vi "PID-Parameter Druckregler einstellen optional.vi"() -> ()   [LabVIEW 2020, in "Erweiterte Konfig.lvlib"]
uses:
  Erweiterte Konfig.lvlib
  Visualisierungs Elemente/Button.ctl
  Visualisierungs Elemente/Zahlen-Eingabefeld.ctl
  Visualisierungs Elemente/Zahlen-Ausgabefeld.ctl
  <vilib>/Utility/miscctls.llb/LVPositionTypeDef.ctl
  cRIO/PC/Aktionen FGV Druckregler.ctl
  cRIO/PC/Kommunikation mit cRIO.lvlib
  Allgemein/allgemeine Sub-VIs.lvlib
  Sprachverwaltung/Sprachverwaltung.lvlib
panel:
  in  "Nach rechts":bool
  in  "Nach links 2":bool
  in  "Nach rechts 2":bool
  in  "Nach links":bool
  in  "Gaskühler Regler -":T1 caption="Ausgang Regler -" format="%#_5g"
  in  "Gaskühler Regler +":T1 caption="Ausgang Regler +" format="%#_5g"
  in  "Gaskühler D":T1 caption="Ausgang D" format="%#_5g"
  in  "Gaskühler I":T1 caption="Ausgang I" format="%#_5g"
  in  "Gaskühler P":T1 caption="Ausgang P" format="%#_5g"
  in  "Gaskühler Regler Toleranz":bool caption="Ausgang Regler Toleranz"
  out "Gaskühler Sollwert":T2 caption="Ausgang Sollwert" format="%.1f"
  out "Gaskühler Istwert":T2 caption="Ausgang Istwert" format="%.1f"
  out "Gaskühler Regler Ausgang":T2 caption="Ausgang Regler Ausgang" format="%.2f"
  out "Gaskühler Analog Ausgang":T2 caption="Ausgang Analog Ausgang" format="%.2f"
  out "Gaskühler Integral":T2 caption="Ausgang Integral" format="%.2f"
  out "Gaskühler Derivative":T2 caption="Ausgang Derivative" format="%.2f"
  out "Gaskühler":sgl[][](graph) caption="Ausgang"
  in  "Druck Kalter Block Regler -":T1 caption="Ausgang Regler -" format="%#_5g"
  in  "Druck Kalter Block Regler +":T1 caption="Ausgang Regler +" format="%#_5g"
  in  "Druck Kalter Block D":T1 caption="Ausgang D" format="%#_5g"
  in  "Druck Kalter Block I":T1 caption="Ausgang I" format="%#_5g"
  in  "Druck Kalter Block P":T1 caption="Ausgang P" format="%#_5g"
  in  "Druck Kalter Block Regler Toleranz":bool caption="Ausgang Regler Toleranz"
  out "Druck Kalter Block Sollwert":T2 caption="Ausgang Sollwert" format="%.1f"
  out "Druck Kalter Block Istwert":T2 caption="Ausgang Istwert" format="%.1f"
  out "Druck Kalter Block Regler Ausgang":T2 caption="Ausgang Regler Ausgang" format="%.2f"
  out "Druck Kalter Block Analog Ausgang":T2 caption="Ausgang Analog Ausgang" format="%.2f"
  out "Druck Kalter Block Integral":T2 caption="Ausgang Integral" format="%.2f"
  out "Druck Kalter Block Derivative":T2 caption="Ausgang Derivative" format="%.2f"
  out "Druck Kalter Block":sgl[][](graph) caption="Ausgang"
  out "Pumpe":sgl[][](graph)
  out "Pumpe Derivative":T2 format="%.2f"
  out "Pumpe Integral":T2 format="%.2f"
  out "Pumpe Analog Ausgang":T2 format="%.2f"
  out "Pumpe Regler Ausgang":T2 format="%.2f"
  out "Pumpe Istwert":T2 format="%.1f"
  out "Pumpe Sollwert":T2 format="%.1f"
  in  "Pumpe Regler -":T1 format="%#_5g"
  in  "Pumpe Regler +":T1 format="%#_5g"
  in  "Pumpe D":T1 format="%#_5g"
  in  "Pumpe I":T1 format="%#_5g"
  in  "Pumpe P":T1 format="%#_5g"
  in  "Pumpe Regler Toleranz":bool
  in  "BEENDEN":T3
  in  "Ausgang Regler -":T1 format="%#_5g"
  in  "Ausgang Regler +":T1 format="%#_5g"
  in  "Ausgang D":T1 format="%#_5g"
  in  "Ausgang I":T1 format="%#_5g"
  in  "Ausgang P":T1 format="%#_5g"
  in  "Ausgang Regler Toleranz":bool
  out "Ausgang Sollwert":T2 format="%.1f"
  out "Ausgang Istwert":T2 format="%.1f"
  out "Ausgang Regler Ausgang":T2 format="%.2f"
  out "Ausgang Analog Ausgang":T2 format="%.2f"
  out "Ausgang Integral":T2 format="%.2f"
  out "Ausgang Derivative":T2 format="%.2f"
  out "Ausgang":sgl[][](graph)
  out "FT-IR":sgl[][](graph)
  out "FT-IR Sollwert":T2 format="%.2f"
  out "FT-IR Istwert":T2 format="%.2f"
  out "FT-IR Regler Ausgang":T2 format="%.2f"
  out "FT-IR Analog Ausgang":T2 format="%.2f"
  out "FT-IR Integral":T2 format="%.2f"
  out "FT-IR Derivative":T2 format="%.2f"
  in  "FT-IR Regler -":T1 format="%#_5g"
  in  "FT-IR Regler +":T1 format="%#_5g"
  in  "FT-IR D":T1 format="%#_5g"
  in  "FT-IR I":T1 format="%#_5g"
  in  "FT-IR P":T1 format="%#_5g"
  in  "FT-IR Regler Toleranz":bool
  # "Parameters Pressure Controller"
  # "Pressure Inlet"
  # "Druck Kalter Block"
  # "Pressure Outlet"
  # "Flow (Pump)"
  # "Gaskühler"
  # "Setpoint:"
  # "Setpoint:"
  # "Setpoint:"
  # "Setpoint:"
  # "Setpoint:"
  # "Intensification KR:"
  # "Intensification KR:"
  # "Intensification KR:"
  # "Intensification KR:"
  # "Intensification KR:"
  # "Actual:"
  # "Actual:"
  # "Actual:"
  # "Actual:"
  # "Actual:"
  # "Reset time TN:"
  # "Reset time TN:"
  # "Reset time TN:"
  # "Reset time TN:"
  # "sec"
  # "sec"
  # "sec"
  # "sec"
  # "Reset time TN:"
  # "sec"
  # "Controller OUT:"
  # "Controller OUT:"
  # "Controller OUT:"
  # "Controller OUT:"
  # "Controller OUT:"
  # "Analog OUT:"
  # "Analog OUT:"
  # "Analog OUT:"
  # "Analog OUT:"
  # "Analog OUT:"
  # "Derivative time TD:"
  # "Derivative time TD:"
  # "Derivative time TD:"
  # "Derivative time TD:"
  # "Derivative time TD:"
  # "sec"
  # "sec"
  # "sec"
  # "sec"
  # "sec"
  # "Intagral Action:"
  # "Intagral Action:"
  # "Intagral Action:"
  # "Intagral Action:"
  # "Intagral Action:"
  # "Derivative Action:"
  # "Derivative Action:"
  # "Derivative Action:"
  # "Derivative Action:"
  # "Derivative Action:"
  # "Contr. tolerance +:"
  # "Contr. tolerance +:"
  # "Contr. tolerance +:"
  # "Contr. tolerance +:"
  # "mbar"
  # "mbar"
  # "Contr. tolerance +:"
  # "l/min"
  # "°C"
  # "mbar"
  # "Contr. tolerance - :"
  # "Contr. tolerance - :"
  # "Contr. tolerance - :"
  # "l/min"
  # "Contr. tolerance - :"
  # "mbar"
  # "mbar"
  # "Contr. tolerance - :"
  # "mbar"
  # "°C"
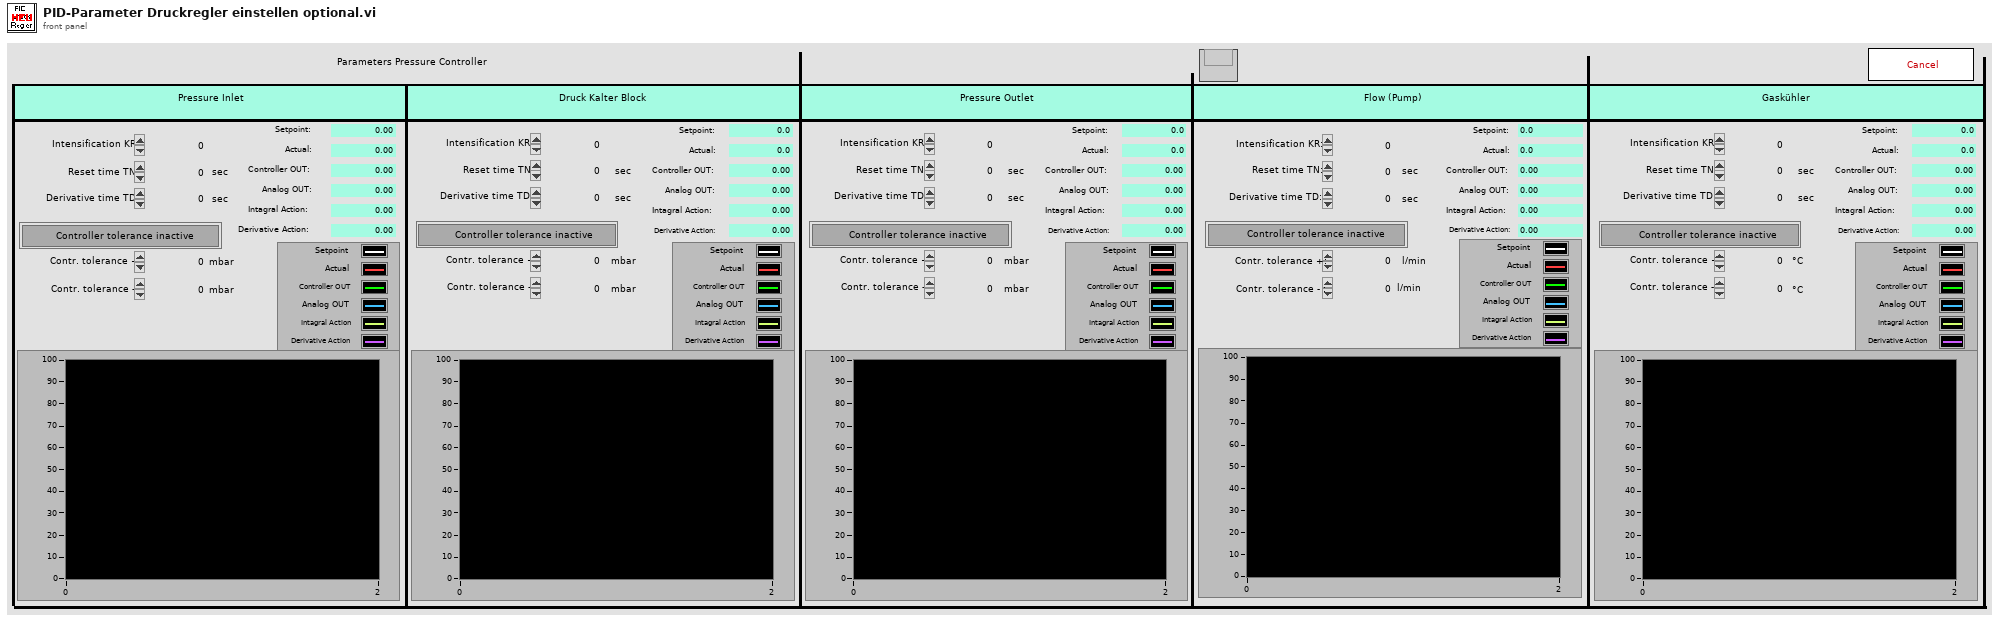
[diagram p1: front panel]
types:
  T1 = typedef "Zahlen-Eingabefeld.ctl" = sgl
  T2 = typedef "Zahlen-Ausgabefeld.ctl" = sgl
  T3 = typedef "Button.ctl" = bool
  T4 = typedef "LVPositionTypeDef.ctl" = cluster{"Left":i32, "Top":i32}
  T5 = typedef "Kommunikation mit cRIO.lvlib/Aktionen FGV Druckregler.ctl" = enum16{"lesen", "Parameter", "Istwerte"}
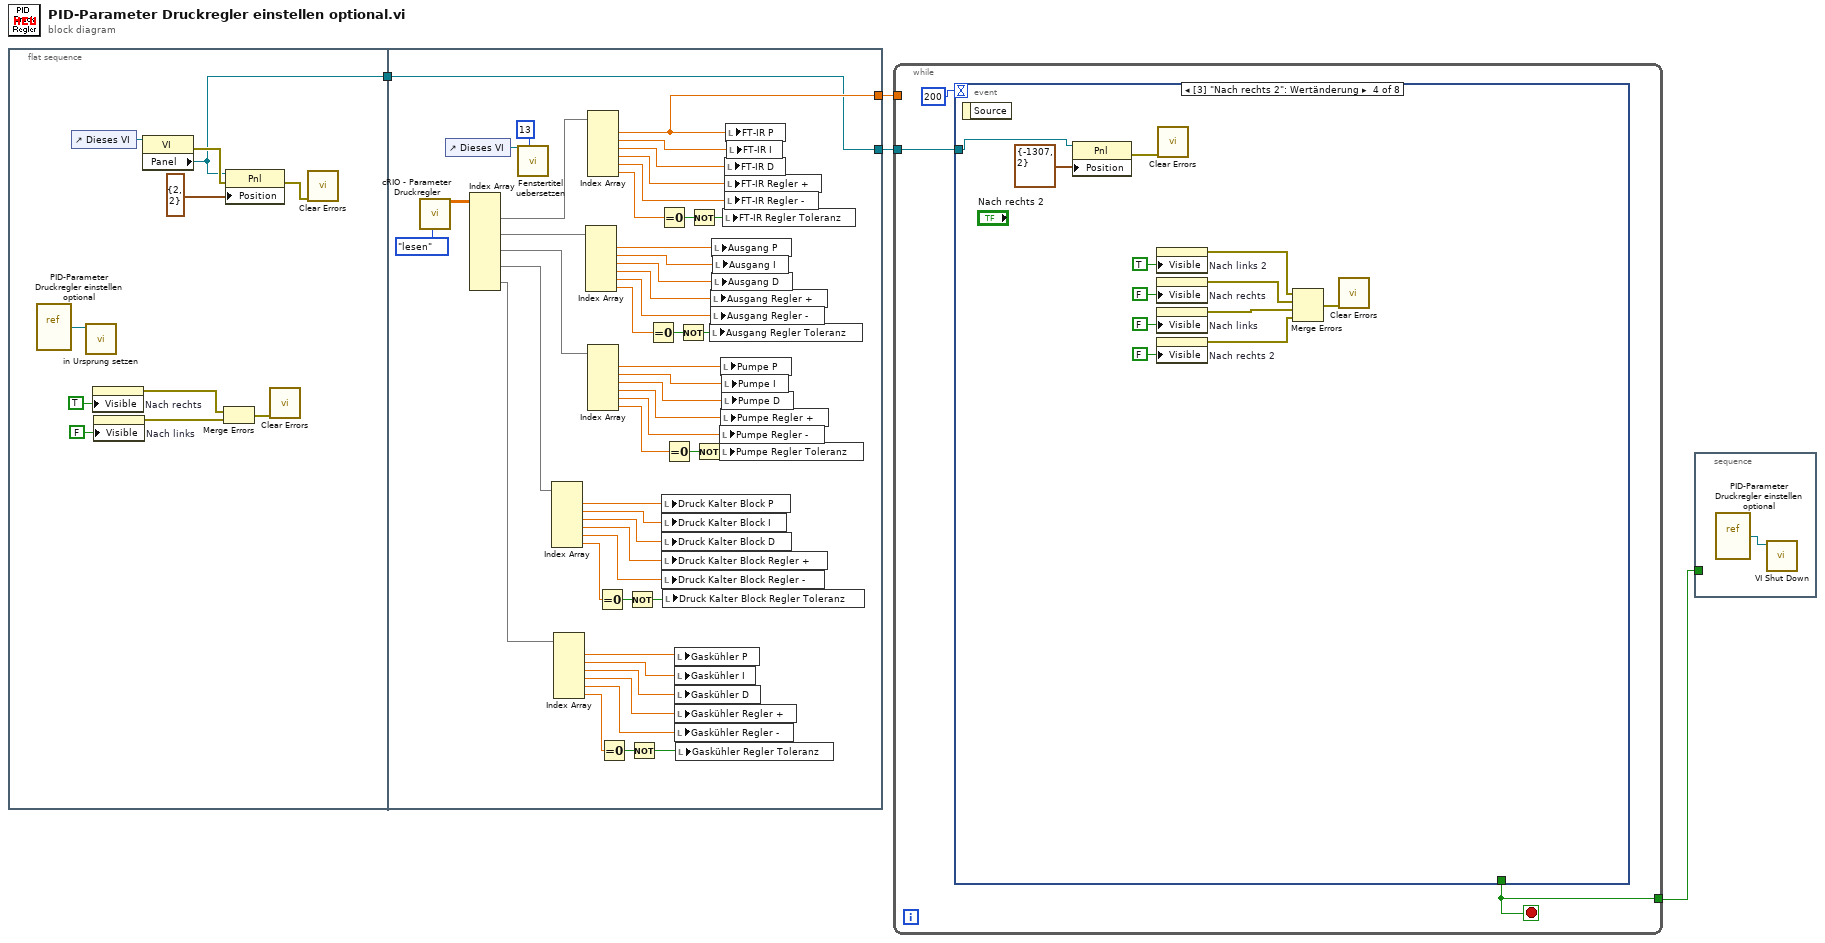
[diagram p0: block diagram]
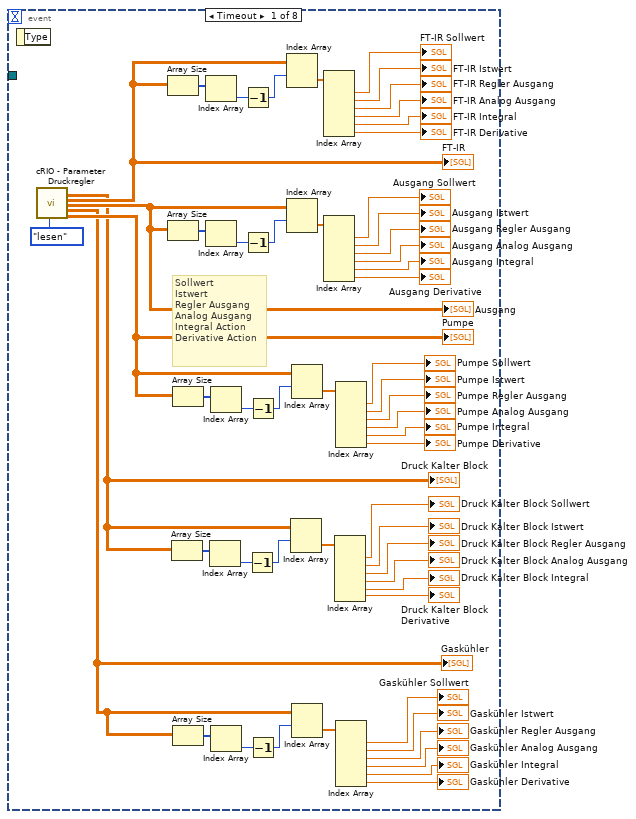
[diagram p2: hidden frame]
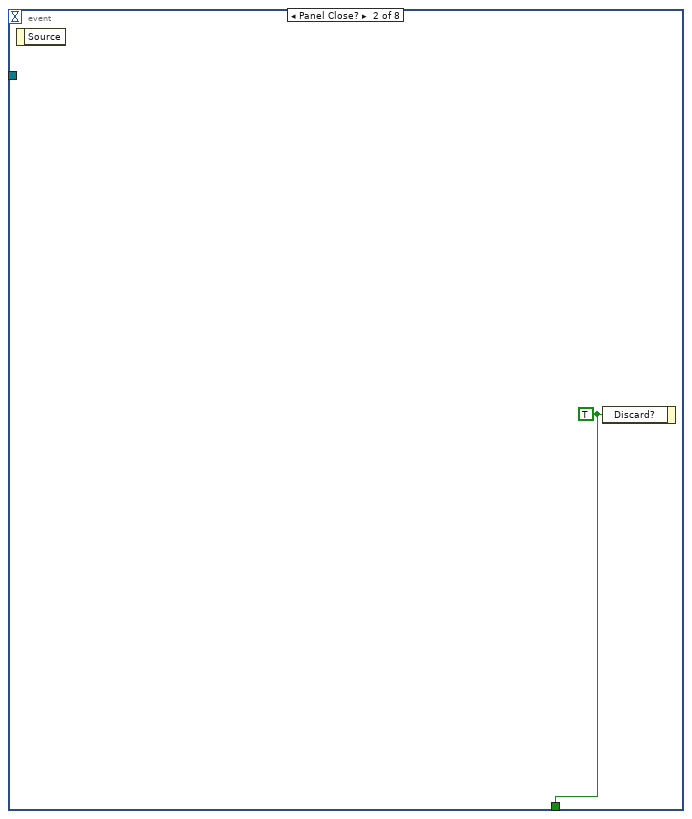
[diagram p3: hidden frame]
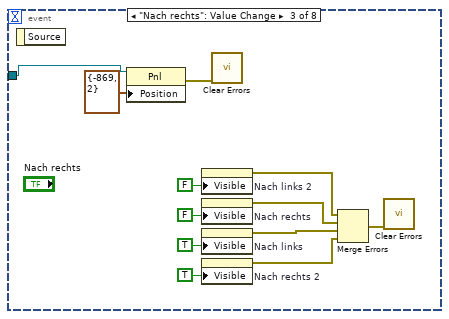
[diagram p4: hidden frame]
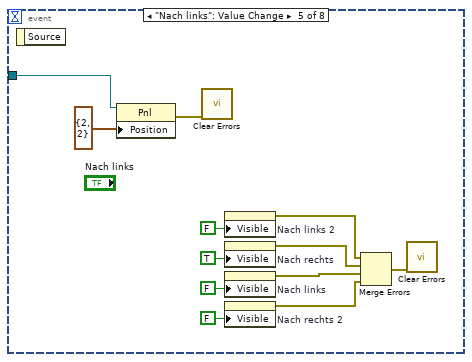
[diagram p5: hidden frame]
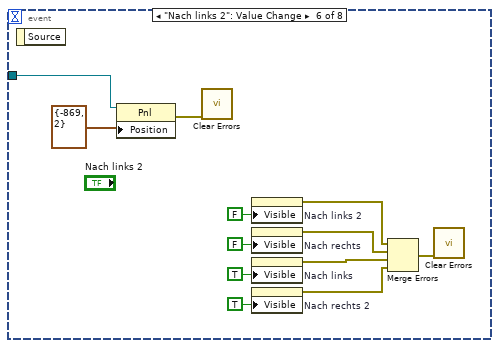
[diagram p6: hidden frame]
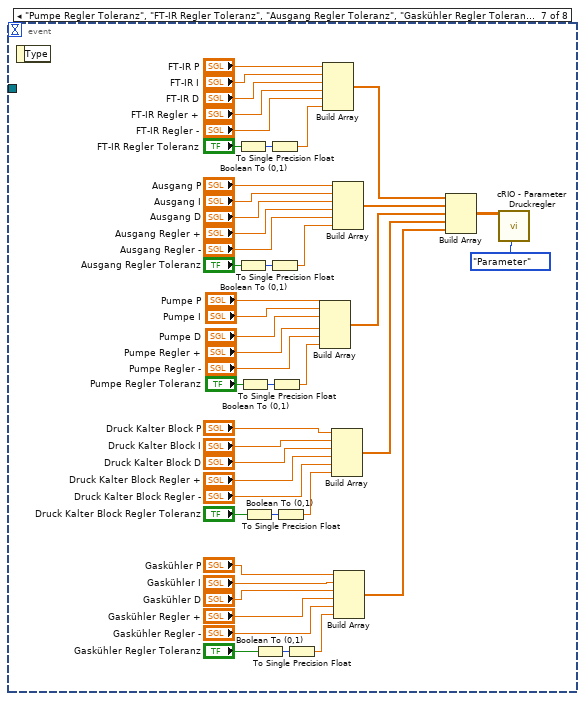
[diagram p7: hidden frame]
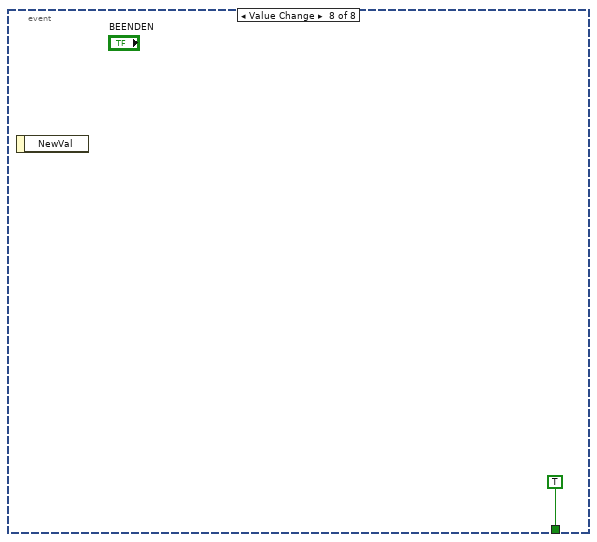
[diagram p8: hidden frame]
diagram:
  n1 = flat-sequence {
    tunnel: [w11] -> w4
    tunnel: [w48] -> w3
    tunnel: w4 -> [w16]
    tunnel: [w16] -> w1
    frame #0 {
      n2 = vi-ref "PID-Parameter Druckregler einstellen optional.vi"() -> (w10:refnum<vi>)
      n3 = control-ref of="Dieses VI"() -> (w15:refnum<vi>)
      n4 = call "in Ursprung setzen.vi"("VI Referenz"=w10) -> ()  [unwired: 11 in]
      n5 = property on="Nach rechts" class="Bool."("Visible"=TRUE ("Sichtbar")) -> (error out=w7:errorcluster)  [unwired: 2 in, 1 out]
      n6 = property on="Nach links" class="Bool."("Visible"=FALSE ("Sichtbar")) -> (error out=w6:errorcluster)  [unwired: 2 in, 1 out]
      n7 = property class="VI"(reference=w15) -> (error out=w13:errorcluster, "Panel"=w11:refnum<vi>)  [unwired: 1 in, 1 out]
      n8 = Merge Errors(w7, w6) -> (w5:errorcluster)
      n9 = property class="Pnl"(reference=w11, error in=w13, "Position"=T4 {"Left"=2, "Top"=2}) -> (error out=w12:errorcluster)  [unwired: 1 out]
      n10 = call <vilib>:"Clear Errors.vi"("error in (no error)"=w5) -> ()  [unwired: 5 in, 2 out]
      n11 = call <vilib>:"Clear Errors.vi"("error in (no error)"=w12) -> ()  [unwired: 5 in, 2 out]
    }
    frame #1 {
      n12 = call "cRIO - Parameter Druckregler.vi"("Aktion"=Aktionen_FGV_Druckregler."lesen") -> ("Parameter Regler"=w59:sgl[][])  [unwired: 9 in, 9 out]
      n13 = control-ref of="Dieses VI"() -> (w36:refnum<vi>)
      n14 = Index Array(array=w59) -> (element #1=w49:sgl[], element #2=w50:sgl[], element #3=w51:sgl[], element #4=w31:sgl[], element #5=w17:sgl[])  [unwired: 10 in]
      n15 = call "Fenstertitel uebersetzen.vi"("Index (Seite)"=13, "Dieses VI"=w36) -> ()  [unwired: 8 in, 2 out]
      n16 = Index Array(array=w31) -> (element #1=w30:sgl, element #2=w29:sgl, element #3=w28:sgl, element #4=w27:sgl, element #5=w26:sgl, element #6=w32:sgl)  [unwired: 6 in]
      n17 = Index Array(array=w17) -> (element #1=w18:sgl, element #2=w19:sgl, element #3=w20:sgl, element #4=w21:sgl, element #5=w22:sgl, element #6=w25:sgl)  [unwired: 6 in]
      n18 = Index Array(array=w50) -> (element #1=w56:sgl, element #2=w55:sgl, element #3=w54:sgl, element #4=w42:sgl, element #5=w41:sgl, element #6=w40:sgl)  [unwired: 6 in]
      n19 = Index Array(array=w49) -> (element #1=w48:sgl, element #2=w58:sgl, element #3=w57:sgl, element #4=w45:sgl, element #5=w44:sgl, element #6=w43:sgl)  [unwired: 6 in]
      n20 = Index Array(array=w51) -> (element #1=w61:sgl, element #2=w65:sgl, element #3=w64:sgl, element #4=w39:sgl, element #5=w38:sgl, element #6=w37:sgl)  [unwired: 6 in]
      n21 = Equal To 0?(x=w32) -> (x = 0?=w34:bool)
      n22 = Equal To 0?(x=w25) -> (x = 0?=w24:bool)
      n23 = Not(x=w34) -> (.not. x?=w33:bool)
      n24 = Not(x=w24) -> (.not. x?=w23:bool)
      n25 = Equal To 0?(x=w40) -> (x = 0?=w53:bool)
      n26 = Equal To 0?(x=w43) -> (x = 0?=w47:bool)
      n27 = local write "Druck Kalter Block P"(w30) -> ()
      n28 = local write "Druck Kalter Block I"(w29) -> ()
      n29 = local write "Druck Kalter Block D"(w28) -> ()
      n30 = local write "Druck Kalter Block Regler +"(w27) -> ()
      n31 = local write "Druck Kalter Block Regler -"(w26) -> ()
      n32 = local write "Druck Kalter Block Regler Toleranz"(w33) -> ()
      n33 = Equal To 0?(x=w37) -> (x = 0?=w63:bool)
      n34 = local write "Gaskühler P"(w18) -> ()
      n35 = local write "Gaskühler I"(w19) -> ()
      n36 = local write "Gaskühler D"(w20) -> ()
      n37 = local write "Gaskühler Regler +"(w21) -> ()
      n38 = local write "Gaskühler Regler -"(w22) -> ()
      n39 = local write "Gaskühler Regler Toleranz"(w23) -> ()
      n40 = Not(x=w53) -> (.not. x?=w52:bool)
      n41 = Not(x=w47) -> (.not. x?=w46:bool)
      n42 = Not(x=w63) -> (.not. x?=w62:bool)
      n43 = local write "Ausgang Regler Toleranz"(w52) -> ()
      n44 = local write "Ausgang Regler +"(w42) -> ()
      n45 = local write "Ausgang Regler -"(w41) -> ()
      n46 = local write "Ausgang P"(w56) -> ()
      n47 = local write "Ausgang D"(w54) -> ()
      n48 = local write "Ausgang I"(w55) -> ()
      n49 = local write "Pumpe Regler -"(w38) -> ()
      n50 = local write "Pumpe Regler Toleranz"(w62) -> ()
      n51 = local write "Pumpe P"(w61) -> ()
      n52 = local write "Pumpe Regler +"(w39) -> ()
      n53 = local write "Pumpe I"(w65) -> ()
      n54 = local write "Pumpe D"(w64) -> ()
      n55 = local write "FT-IR Regler Toleranz"(w46) -> ()
      n56 = local write "FT-IR D"(w57) -> ()
      n57 = local write "FT-IR Regler +"(w45) -> ()
      n58 = local write "FT-IR Regler -"(w44) -> ()
      n59 = local write "FT-IR P"(w48) -> ()
      n60 = local write "FT-IR I"(w58) -> ()
    }
  }
  n61 = while {
    tunnel: w3 -> [_]
    tunnel: [w67] -> w2
    tunnel: w1 -> [w66]
    stop <- w67 stop-if-true
    n62 = event shown="[3] \"Nach rechts 2\": Wertänderung" {
      selector: _ -> [_ _ _ _ _ _ _ _]
      dyn-events: _ -> [_ _ _ _ _ _ _ _]
      timeout: 200 -> [_ _ _ _ _ _ _ _]
      tunnel: [_ w125 _ _ _ _ _ TRUE ("ABBRECHEN")] -> w67
      tunnel: w66 -> [_ _ w136 w148 w159 w171 _ _]
      event Timeout {
        # "Sollwert\nIstwert\nRegler Ausgang\nAnalog Ausgang\nIntegral Action\nDerivative Action"
        n63 = event-data() -> ()  [unwired: 1 in, 1 out]
        n64 = call "cRIO - Parameter Druckregler.vi"("Aktion"=Aktionen_FGV_Druckregler."lesen") -> ("Istwerte Regler Druck PMA"=w76:sgl[][], "Istwerte Regler FT-IR"=w103:sgl[][], "Istwerte Regler Ausgang"=w102:sgl[][], "Istwerte Regler NDIR"=w74:sgl[][], "Istwerte Regler Filterblock"=w92:sgl[][])  [unwired: 9 in, 5 out]
        "FT-IR" <- w103
        "Ausgang" <- w102
        "Pumpe" <- w92
        "Druck Kalter Block" <- w76
        "Gaskühler" <- w74
        n65 = Array Size(array=w103) -> (size(s)=w120:i32[])
        n66 = Array Size(array=w102) -> (size(s)=w119:i32[])
        n67 = Array Size(array=w76) -> (size(s)=w87:i32[])
        n68 = Array Size(array=w92) -> (size(s)=w96:i32[])
        n69 = Array Size(array=w74) -> (size(s)=w86:i32[])
        n70 = Index Array(array=w120) -> (element=w121:i32)  [unwired: 1 in]
        n71 = Index Array(array=w119) -> (element=w118:i32)  [unwired: 1 in]
        n72 = Index Array(array=w87) -> (element=w88:i32)  [unwired: 1 in]
        n73 = Index Array(array=w96) -> (element=w95:i32)  [unwired: 1 in]
        n74 = Index Array(array=w86) -> (element=w85:i32)  [unwired: 1 in]
        n75 = Decrement(x=w121) -> (x-1=w122:i32)
        n76 = Decrement(x=w118) -> (x-1=w117:i32)
        n77 = Decrement(x=w88) -> (x-1=w89:i32)
        n78 = Decrement(x=w95) -> (x-1=w94:i32)
        n79 = Decrement(x=w85) -> (x-1=w84:i32)
        n80 = Index Array(array=w103, index (row)=w122) -> (element=w123:sgl[])  [unwired: 1 in]
        n81 = Index Array(array=w102, index (row)=w117) -> (element=w116:sgl[])  [unwired: 1 in]
        n82 = Index Array(array=w76, index (row)=w89) -> (element=w90:sgl[])  [unwired: 1 in]
        n83 = Index Array(array=w92, index (row)=w94) -> (element=w93:sgl[])  [unwired: 1 in]
        n84 = Index Array(array=w74, index (row)=w84) -> (element=w83:sgl[])  [unwired: 1 in]
        n85 = Index Array(array=w123) -> (element #1=→"FT-IR Sollwert":sgl, element #2=→"FT-IR Istwert":sgl, element #3=→"FT-IR Regler Ausgang":sgl, element #4=→"FT-IR Analog Ausgang":sgl, element #5=→"FT-IR Integral":sgl, element #6=→"FT-IR Derivative":sgl)  [unwired: 6 in]
        n86 = Index Array(array=w116) -> (element #1=→"Ausgang Sollwert":sgl, element #2=→"Ausgang Istwert":sgl, element #3=→"Ausgang Regler Ausgang":sgl, element #4=→"Ausgang Analog Ausgang":sgl, element #5=→"Ausgang Integral":sgl, element #6=→"Ausgang Derivative":sgl)  [unwired: 6 in]
        n87 = Index Array(array=w90) -> (element #1=→"Druck Kalter Block Sollwert":sgl, element #2=→"Druck Kalter Block Istwert":sgl, element #3=→"Druck Kalter Block Regler Ausgang":sgl, element #4=→"Druck Kalter Block Analog Ausgang":sgl, element #5=→"Druck Kalter Block Integral":sgl, element #6=→"Druck Kalter Block Derivative":sgl)  [unwired: 6 in]
        n88 = Index Array(array=w93) -> (element #1=→"Pumpe Sollwert":sgl, element #2=→"Pumpe Istwert":sgl, element #3=→"Pumpe Regler Ausgang":sgl, element #4=→"Pumpe Analog Ausgang":sgl, element #5=→"Pumpe Integral":sgl, element #6=→"Pumpe Derivative":sgl)  [unwired: 6 in]
        n89 = Index Array(array=w83) -> (element #1=→"Gaskühler Sollwert":sgl, element #2=→"Gaskühler Istwert":sgl, element #3=→"Gaskühler Regler Ausgang":sgl, element #4=→"Gaskühler Analog Ausgang":sgl, element #5=→"Gaskühler Integral":sgl, element #6=→"Gaskühler Derivative":sgl)  [unwired: 6 in]
      }
      event Panel Close? {
        w125 = TRUE ("Verwerfen?")
        n90 = event-data() -> ()  [unwired: 1 in, 1 out]
        n91 = event-data("Discard?"=w125) -> ()  [unwired: 1 in, 1 out]
      }
      event "Nach rechts": Value Change {
        n92 = event-data() -> ()  [unwired: 1 in, 1 out]
        n93 = property class="Pnl"(reference=w136, "Position"=T4 {"Left"=-869, "Top"=2}) -> (error out=w135:errorcluster)  [unwired: 1 in, 1 out]
        n94 = property on="Nach links 2" class="Bool."("Visible"=FALSE ("Sichtbar")) -> (error out=w130:errorcluster)  [unwired: 2 in, 1 out]
        n95 = property on="Nach rechts" class="Bool."("Visible"=FALSE ("Sichtbar")) -> (error out=w132:errorcluster)  [unwired: 2 in, 1 out]
        n96 = property on="Nach links" class="Bool."("Visible"=TRUE ("Sichtbar")) -> (error out=w133:errorcluster)  [unwired: 2 in, 1 out]
        n97 = property on="Nach rechts 2" class="Bool."("Visible"=TRUE ("Sichtbar")) -> (error out=w131:errorcluster)  [unwired: 2 in, 1 out]
        n98 = call <vilib>:"Clear Errors.vi"("error in (no error)"=w135) -> ()  [unwired: 5 in, 2 out]
        n99 = Merge Errors(w130, w132, w133, w131) -> (w134:errorcluster)
        n100 = call <vilib>:"Clear Errors.vi"("error in (no error)"=w134) -> ()  [unwired: 5 in, 2 out]
      }
      event "Nach rechts 2": Value Change {
        n101 = event-data() -> ()  [unwired: 1 in, 1 out]
        n102 = property class="Pnl"(reference=w148, "Position"=T4 {"Left"=-1307, "Top"=2}) -> (error out=w147:errorcluster)  [unwired: 1 in, 1 out]
        n103 = property on="Nach links 2" class="Bool."("Visible"=TRUE ("Sichtbar")) -> (error out=w142:errorcluster)  [unwired: 2 in, 1 out]
        n104 = property on="Nach rechts" class="Bool."("Visible"=FALSE ("Sichtbar")) -> (error out=w144:errorcluster)  [unwired: 2 in, 1 out]
        n105 = property on="Nach links" class="Bool."("Visible"=FALSE ("Sichtbar")) -> (error out=w145:errorcluster)  [unwired: 2 in, 1 out]
        n106 = property on="Nach rechts 2" class="Bool."("Visible"=FALSE ("Sichtbar")) -> (error out=w143:errorcluster)  [unwired: 2 in, 1 out]
        n107 = call <vilib>:"Clear Errors.vi"("error in (no error)"=w147) -> ()  [unwired: 5 in, 2 out]
        n108 = Merge Errors(w142, w144, w145, w143) -> (w146:errorcluster)
        n109 = call <vilib>:"Clear Errors.vi"("error in (no error)"=w146) -> ()  [unwired: 5 in, 2 out]
      }
      event "Nach links": Value Change {
        n110 = event-data() -> ()  [unwired: 1 in, 1 out]
        n111 = property class="Pnl"(reference=w159, "Position"=T4 {"Left"=2, "Top"=2}) -> (error out=w160:errorcluster)  [unwired: 1 in, 1 out]
        n112 = call <vilib>:"Clear Errors.vi"("error in (no error)"=w160) -> ()  [unwired: 5 in, 2 out]
        n113 = property on="Nach links 2" class="Bool."("Visible"=FALSE ("Sichtbar")) -> (error out=w154:errorcluster)  [unwired: 2 in, 1 out]
        n114 = property on="Nach rechts" class="Bool."("Visible"=TRUE ("Sichtbar")) -> (error out=w156:errorcluster)  [unwired: 2 in, 1 out]
        n115 = property on="Nach links" class="Bool."("Visible"=FALSE ("Sichtbar")) -> (error out=w157:errorcluster)  [unwired: 2 in, 1 out]
        n116 = property on="Nach rechts 2" class="Bool."("Visible"=FALSE ("Sichtbar")) -> (error out=w155:errorcluster)  [unwired: 2 in, 1 out]
        n117 = Merge Errors(w154, w156, w157, w155) -> (w158:errorcluster)
        n118 = call <vilib>:"Clear Errors.vi"("error in (no error)"=w158) -> ()  [unwired: 5 in, 2 out]
      }
      event "Nach links 2": Value Change {
        n119 = event-data() -> ()  [unwired: 1 in, 1 out]
        n120 = property class="Pnl"(reference=w171, "Position"=T4 {"Left"=-869, "Top"=2}) -> (error out=w172:errorcluster)  [unwired: 1 in, 1 out]
        n121 = call <vilib>:"Clear Errors.vi"("error in (no error)"=w172) -> ()  [unwired: 5 in, 2 out]
        n122 = property on="Nach links 2" class="Bool."("Visible"=FALSE ("Sichtbar")) -> (error out=w166:errorcluster)  [unwired: 2 in, 1 out]
        n123 = property on="Nach rechts" class="Bool."("Visible"=FALSE ("Sichtbar")) -> (error out=w168:errorcluster)  [unwired: 2 in, 1 out]
        n124 = property on="Nach links" class="Bool."("Visible"=TRUE ("Sichtbar")) -> (error out=w169:errorcluster)  [unwired: 2 in, 1 out]
        n125 = property on="Nach rechts 2" class="Bool."("Visible"=TRUE ("Sichtbar")) -> (error out=w167:errorcluster)  [unwired: 2 in, 1 out]
        n126 = Merge Errors(w166, w168, w169, w167) -> (w170:errorcluster)
        n127 = call <vilib>:"Clear Errors.vi"("error in (no error)"=w170) -> ()  [unwired: 5 in, 2 out]
      }
      event "Pumpe Regler Toleranz", "FT-IR Regler Toleranz", "Ausgang Regler Toleranz", "Gaskühler Regler Toleranz", "Druck Kalter Block Regler Toleranz": Value Change {
        n128 = event-data() -> ()  [unwired: 1 in, 1 out]
        n129 = Boolean To (0,1)(Boolean="FT-IR Regler Toleranz") -> (0, 1=w220:i16)
        n130 = Boolean To (0,1)(Boolean="Ausgang Regler Toleranz") -> (0, 1=w214:i16)
        n131 = Boolean To (0,1)(Boolean="Pumpe Regler Toleranz") -> (0, 1=w206:i16)
        n132 = Boolean To (0,1)(Boolean="Druck Kalter Block Regler Toleranz") -> (0, 1=w191:i16)
        n133 = Boolean To (0,1)(Boolean="Gaskühler Regler Toleranz") -> (0, 1=w181:i16)
        n134 = To Single Precision Float(number=w220) -> (single precision float=w198:sgl)
        n135 = To Single Precision Float(number=w214) -> (single precision float=w197:sgl)
        n136 = To Single Precision Float(number=w206) -> (single precision float=w192:sgl)
        n137 = To Single Precision Float(number=w191) -> (single precision float=w189:sgl)
        n138 = To Single Precision Float(number=w181) -> (single precision float=w179:sgl)
        n139 = Build Array("Pumpe P", "Pumpe I", "Pumpe D", "Pumpe Regler +", "Pumpe Regler -", w192) -> (w201:T1[])
        n140 = Build Array("FT-IR P", "FT-IR I", "FT-IR D", "FT-IR Regler +", "FT-IR Regler -", w198) -> (w209:T1[])
        n141 = Build Array("Druck Kalter Block P", "Druck Kalter Block I", "Druck Kalter Block D", "Druck Kalter Block Regler +", "Druck Kalter Block Regler -", w189) -> (w183:T1[])
        n142 = Build Array("Ausgang P", "Ausgang I", "Ausgang D", "Ausgang Regler +", "Ausgang Regler -", w197) -> (w208:T1[])
        n143 = Build Array("Gaskühler P", "Gaskühler I", "Gaskühler D", "Gaskühler Regler +", "Gaskühler Regler -", w179) -> (w182:T1[])
        n144 = Build Array(w209, w208, w201, w183, w182) -> (w207:T1[][])
        n145 = call "cRIO - Parameter Druckregler.vi"("Parameter Regler"=w207, "Aktion"=Aktionen_FGV_Druckregler."Parameter") -> ()  [unwired: 8 in, 10 out]
      }
      event Value Change {
        n146 = event-data() -> ()  [unwired: 1 in, 1 out]
      }
    }
  }
  n147 = stacked-sequence {
    tunnel: w2 -> [_]
    frame #0 {
      n148 = vi-ref "PID-Parameter Druckregler einstellen optional.vi"() -> (w222:refnum<vi>)
      n149 = call "VI Shut Down.vi"("VI Referenz"=w222) -> ()  [unwired: 11 in]
    }
  }
